vi "PH_DeformableMirror.SetAllChannels.vi"(0 "i ref in":refnum<vi>, 2 "Voltages":dbl[](array[numeric]), 5 "error in":errorcluster) -> (14 "i ref out":refnum<vi>, 19 "error out":errorcluster)   [LabVIEW 2014, in "PH_DeformableMirror.lvlib"]
uses:
  PH_DeformableMirror.lvlib
  instr.lib/dmdriver/DMirrorBase/DMirrorBase.lvclass
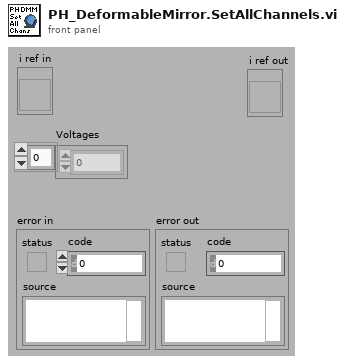
[diagram p1: front panel]
types:
  T1 = typedef "PH_DeformableMirror.lvlib/PH_DeformableMirror.i attribute.ctl" = cluster{"DMirror.lvlib:DMirrorBase.lvclass":refnum<class "DMirrorBase.lvclass">, "Device error":errorcluster, "GUI Refs":cluster{"Delete":refnum<vi>, "Device Error":refnum<vi>, "HV on":refnum<vi>, "Channel":refnum<vi>, "Voltage":refnum<vi>, "Channel Voltages":refnum<vi>}}
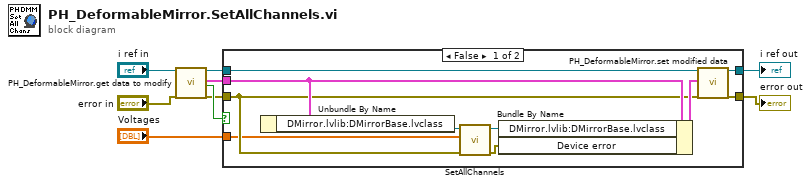
[diagram p0: block diagram]
diagram:
  n1 = call "PH_DeformableMirror.get data to modify.vi"("i ref in"="i ref in", "error in (no error)"="error in") -> ("i ref out"=w5:refnum<vi>, "i attribute"=w2:T1, "timed out"=w9:bool, "error out"=w3:errorcluster)  [unwired: 14 in]
  n2 = case shown="False" w9 {
    tunnel: [w19 w21] -> w7
    tunnel: w5 -> [w18 w21]
    tunnel: [w17 w20] -> w6
    tunnel: w3 -> [w11 w20]
    tunnel: w2 -> [w16 _]
    tunnel: "Voltages" -> [w10 _]
    frame False {
      n3 = Unbundle By Name(w16) -> ("DMirror.lvlib:DMirrorBase.lvclass"=w15:refnum<class "DMirrorBase.lvclass">)
      n4 = call-dynamic "SetAllChannels.vi"("error in (no error)"=w11, "Voltages"=w10, "DMirrorBase in"=w15) -> ("error out"=w12:errorcluster, "DMirrorBase out"=w13:refnum<class "DMirrorBase.lvclass">)  [unwired: 7 in]
      n5 = Bundle By Name(cluster=w16, "DMirror.lvlib:DMirrorBase.lvclass"=w13, "Device error"=w12) -> (w14:T1)
      n6 = call "PH_DeformableMirror.set modified data.vi"("i ref in"=w18, "i attribute"=w14, "error in (no error)"=w11) -> ("i ref out"=w19:refnum<vi>, "error out"=w17:errorcluster)  [unwired: 15 in]
    }
    frame True {
    }
  }
  "error out" <- w6
  "i ref out" <- w7
